vi "MoveCW.vi"(8 "error in (no error)":errorcluster, 11 "Data in":T1) -> (0 "error out":errorcluster, 3 "Data out":T1)   [LabVIEW 2019, in "ManualMode.lvlib"]
uses:
  ManualMode.lvlib
  Cluster - ManualModeData.ctl
  MainController/Cluster - HardwareConfiguration.ctl
  Mark10 API/WriteSpeed.vi
  Mark10 API/WriteCWTravelLimit.vi
  Mark10 API/Mark 10 TSTM-DC.lvlib
  Utilites/Utilities.lvlib
  EventLogger/EventLogger.lvlib
  MainController/MainController.lvlib
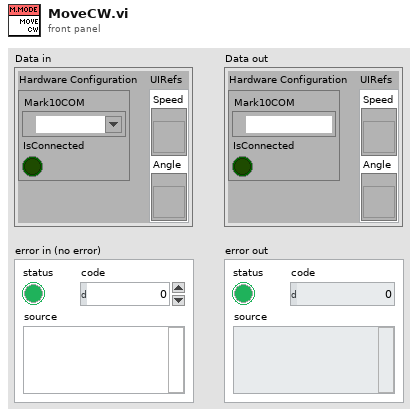
[diagram p1: front panel]
types:
  T1 = typedef "ManualMode.lvlib/Cluster - ManualModeData.ctl" = cluster{"Hardware Configuration":T2, "UIRefs":cluster{"Speed":refnum<vi>, "Angle":refnum<vi>}}
  T2 = typedef "MainController.lvlib/Cluster - HardwareConfiguration.ctl" = cluster{"Mark10COM":refnum<visa-resource-name>, "IsConnected":bool}
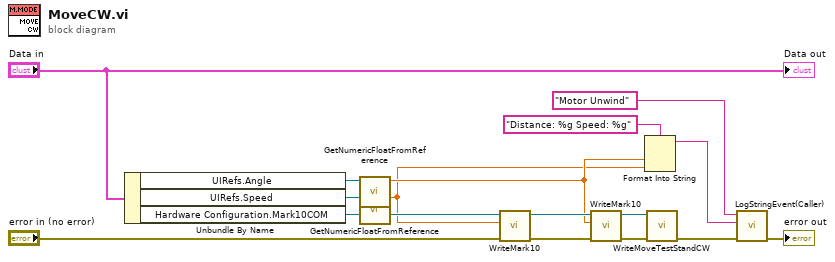
[diagram p0: block diagram]
diagram:
  n1 = Unbundle By Name("Data in") -> ("UIRefs.Angle"=w8:refnum<vi>, "UIRefs.Speed"=w7:refnum<vi>, "Hardware Configuration.Mark10COM"=w13:refnum<visa-resource-name>)
  n2 = call "GetNumericFloatFromReference.vi"("reference"=w8) -> ("Value"=w3:dbl)  [unwired: 9 in, 1 out]
  n3 = call "GetNumericFloatFromReference.vi"("reference"=w7) -> ("Value"=w2:dbl)  [unwired: 9 in, 1 out]
  n4 = call-poly "WriteMark10.vi"("error in"="error in (no error)", "Speed"=w2, "VISA resource name"=w13) -> ("error out"=w12:errorcluster, "VISA resource name out"=w11:refnum<visa-resource-name>)  [unwired: 7 in]
  n5 = call-poly "WriteMark10.vi"("error in"=w12, "CWTravelLimit"=w3, "VISA resource name"=w11) -> ("error out"=w10:errorcluster, "VISA resource name out"=w9:refnum<visa-resource-name>)  [unwired: 7 in]
  n6 = Format Into String(format string="Distance: %g Speed: %g", w3, w2) -> (resulting string=w1:string)  [unwired: 2 in, 1 out]
  n7 = call "WriteMoveTestStandCW.vi"("error in"=w10, "VISA resource name"=w9) -> ("error out"=w15:errorcluster)  [unwired: 8 in, 1 out]
  n8 = call "LogStringEvent(Caller).vi"("Error In"=w15, "Data"=w1, "Field"="Motor Unwind") -> ("Error Out"=→"error out":errorcluster)  [unwired: 8 in]
  "Data out" <- "Data in"
